vi "New Queue Log.vi"(6 "queue (default: new)":refnum<queue>, 7 "context":string, 8 "error in (no error)":errorcluster, 10 "level":T1 items=["OFF"=0, "FATAL"=100, "ERROR"=200, "WARN"=300, "INFO"=400, "DEBUG"=500, "TRACE"=600, "ALL"=65535]) -> (0 "error out":errorcluster, 1 "queue out":refnum<queue>, 3 "Queue Log Provider":refnum<data-value>)   [LabVIEW 2019, in "Utility API.lvlib" / "Queue Log Provider.lvclass"]
doc: "<b>Description</b> Create a new queue-based logging provider. If you do not wire an input queue, a new string-typed queue reference will be created and returned. \n\n<b>Inputs</b>\n<b>context</b>: The default context of the logger. The default context of the logger can be changed using 'Set Context'.\n<b>level</b>: The default logging level of the logger. This level can be chaged using 'Set Log Level'.\n<b>queue</b>: A string-typed queue reference. If you do not wire this input, a new queue reference will be created and returned.\n\n<b>Outputs</b>\n<b>Queue Log Provider</b>: A new logger provider instance.\n<b>queue out</b>: A duplicate of the input queue reference, or a new queue reference if the input was an invalid reference.\n\nBSD 3-Clause License\n\nCopyright (c) 2021, TauTerra, LLC\nAll rights reserved.\n\nRedistribution and use in source and binary forms, with or without\nmodification, are permitted provided that the following conditions are met:\n\n1. Redistributions of source code must retain the above copyright notice, this\n list of conditions and the following disclaimer.\n\n2. Redistributions in binary form must reproduce the above copyright notice,\n this list of conditions and the following disclaimer in the documentation\n and/or other materials provided with the distribution.\n\n3. Neither the name of the copyright holder nor the names of its\n contributors may be used to endorse or promote products derived from\n this software without specific prior written permission.\n\nTHIS SOFTWARE IS PROVIDED BY THE COPYRIGHT HOLDERS AND CONTRIBUTORS \"AS IS\"\nAND ANY EXPRESS OR IMPLIED WARRANTIES, INCLUDING, BUT NOT LIMITED TO, THE\nIMPLIED WARRANTIES OF MERCHANTABILITY AND FITNESS FOR A PARTICULAR PURPOSE ARE\nDISCLAIMED. IN NO EVENT SHALL THE COPYRIGHT HOLDER OR CONTRIBUTORS BE LIABLE\nFOR ANY DIRECT, INDIRECT, INCIDENTAL, SPECIAL, EXEMPLARY, OR CONSEQUENTIAL\nDAMAGES (INCLUDING, BUT NOT LIMITED TO, PROCUREMENT OF SUBSTITUTE GOODS OR\nSERVICES; LOSS OF USE, DATA, OR PROFITS; OR BUSINESS INTERRUPTION) HOWEVER\nCAUSED AND ON ANY THEORY OF LIABILITY, WHETHER IN CONTRACT, STRICT LIABILITY,\nOR TORT (INCLUDING NEGLIGENCE OR OTHERWISE) ARISING IN ANY WAY OUT OF THE USE\nOF THIS SOFTWARE, EVEN IF ADVISED OF THE POSSIBILITY OF SUCH DAMAGE."
uses:
  Queue Log Provider.lvclass
  Log Service/public/level.ctl
  impl/log_message.ctl
  Queue Log Provider.lvclass/Queue Log Provider.ctl
  Log Service/Log Service.lvclass
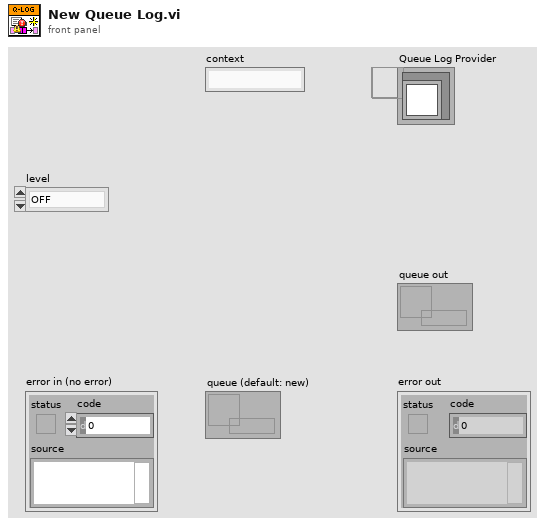
[diagram p1: front panel]
types:
  T1 = typedef "Utility API.lvlib/Log Service.lvclass/level.ctl" = u16
  T2 = typedef "Utility API.lvlib/Queue Log Provider.lvclass/log_message.ctl" = cluster{"Time Stamp":timestamp, "level":T1, "context":string, "message":string}
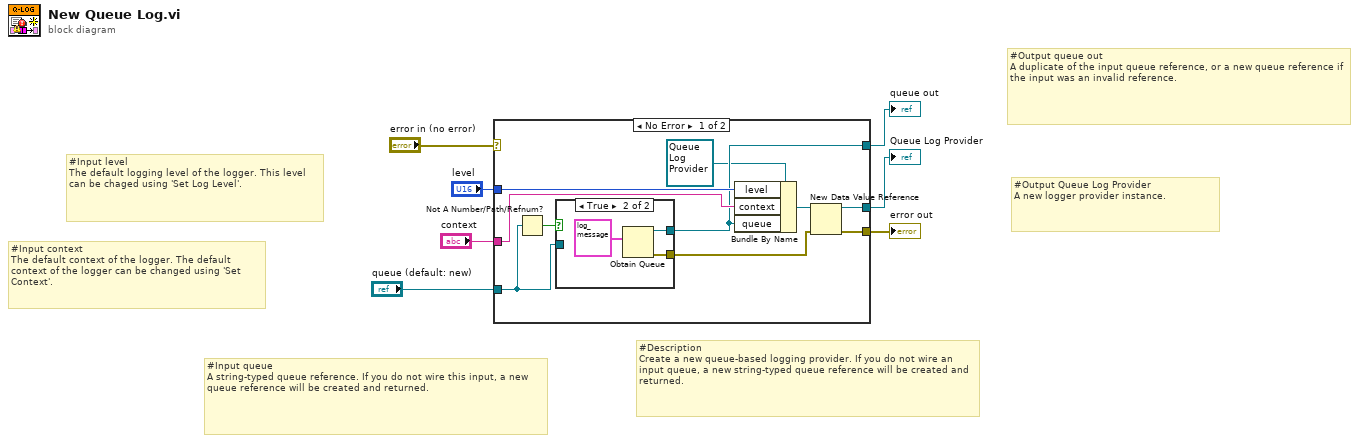
[diagram p0: block diagram]
diagram:
  # "#Input context\nThe default context of the logger. The default context of the logger can be changed using 'Set Context'."
  # "#Input level\nThe default logging level of the logger. This level can be chaged using 'Set Log Level'."
  # "#Output Queue Log Provider\nA new logger provider instance."
  # "#Output queue out\nA duplicate of the input queue reference, or a new queue reference if the input was an invalid reference."
  # "#Input queue\nA string-typed queue reference. If you do not wire this input, a new queue reference will be created and returned."
  # "#Description\nCreate a new queue-based logging provider. If you do not wire an input queue, a new string-typed queue reference will be created and returned."
  n1 = case shown="No Error" "error in (no error)" {
    selector: "error in (no error)" -> [_ w23]
    tunnel: [w12 w23] -> w6
    tunnel: [w9 _] -> w5
    tunnel: "queue (default: new)" -> [w14 w22]
    tunnel: "context" -> [w16 _]
    tunnel: "level" -> [w15 _]
    tunnel: [w13 w22] -> w1
    frame No Error {
      n2 = Not A Number/Path/Refnum?(number/path/refnum=w14) -> (NaN/Path/Refnum?=w17:bool)
      n3 = case shown="True" w17 {
        tunnel: [w18 w20] -> w13
        tunnel: w14 -> [w18 _]
        tunnel: [_ w19] -> w11
        frame False {
        }
        frame True {
          n4 = Obtain Queue(element data type=T2 {"Time Stamp"=timestamp(0 s since 1904-01-01), "level"=0, "context"="", "message"=""} ("message")) -> (queue out=w20:refnum<queue>, error out=w19:errorcluster)  [unwired: 4 in, 1 out]
        }
      }
      n5 = Bundle By Name(cluster=refnum<class "Queue Log Provider.lvclass"> refnum ("Queue Log Provider in"), "level"=w15, "context"=w16, "queue"=w13) -> (w10:refnum<class "Queue Log Provider.lvclass">)
      n6 = New Data Value Reference(data value=w10, error in=w11) -> (data value reference=w9:refnum<data-value>, error out=w12:errorcluster)
    }
    frame Error {
    }
  }
  "error out" <- w6
  "Queue Log Provider" <- w5
  "queue out" <- w1
